vi "Get Current Hour Data ver2.vi"(9 "Shift":string, 10 "Total Hours per Shift":i32=12, 11 "Refnum in":T1) -> (0 "Current Hour Actual":u32, 1 "Hour Index":i32, 2 "Shift Hour Data":u32[][](array[numeric]), 3 "Refnum Out":T1, 4 "Current Hour Target":u32)   [LabVIEW 2018]
uses:
  <vilib>/Utility/config.llb/Config Data RefNum.ctl
  <vilib>/Utility/config.llb/Read Key (String).vi
  <vilib>/Utility/config.llb/NI_LVConfig.lvlib
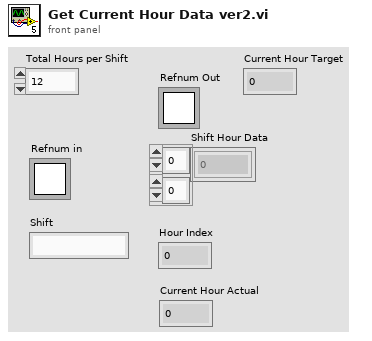
[diagram p1: front panel]
types:
  T1 = typedef "NI_LVConfig.lvlib/Config Data RefNum.ctl" = refnum<k1>
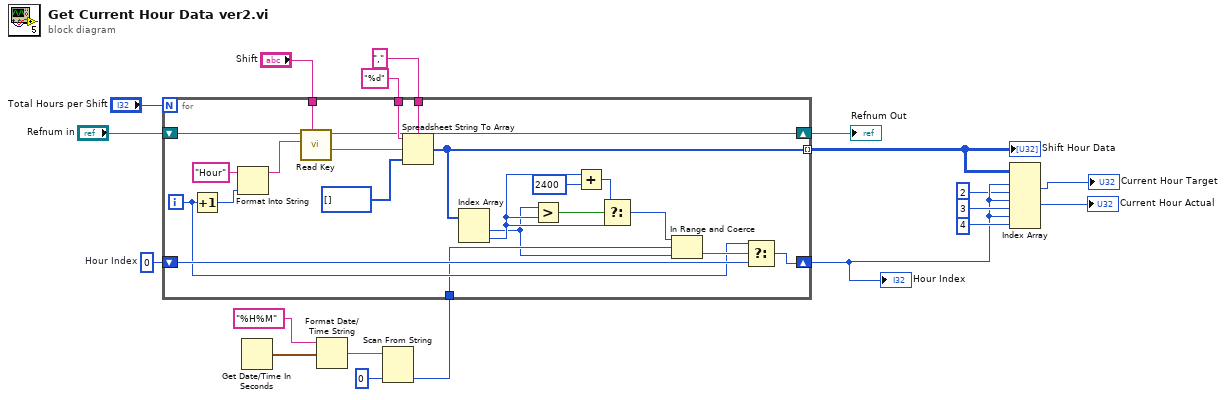
[diagram p0: block diagram]
diagram:
  w16 = 0  # Hour Index
  n1 = Get Date/Time In Seconds() -> (seconds since 1Jan1904=w4:timestamp)
  n2 = Format Date/Time String(time format string (%c)="%H%M", seconds (now)=w4) -> (date/time string=w11:string)  [unwired: 1 in]
  n3 = Scan From String(input string=w11, default 1=u32 0) -> (output 1=w15:u32)  [unwired: 3 in, 3 out]
  n4 = for {
    N: "Total Hours per Shift" -> [_]
    tunnel: "Shift" -> [w41]
    tunnel: [w27] -> w19 mode=indexing
    tunnel: "," ("delimiter (Tab)") -> [w34]
    tunnel: "%d" ("format string") -> [w33]
    tunnel: w15 -> [w28]
    shift-right: [w32] -> w6
    shift-left: w16 -> [w31]
    shift-right: [w26] -> w8
    shift-left: "Refnum in" -> [w40]
    i -> [w29]
    n5 = Increment(x=w29) -> (x+1=w37:i32)
    n6 = Format Into String(initial string="Hour", w37) -> (resulting string=w39:string)  [unwired: 2 in, 1 out]
    n7 = call-poly <vilib>:"Read Key.vi"("section"=w41, "key"=w39, "refnum"=w40) -> ("value"=w36:string, "refnum out"=w26:T1)  [unwired: 5 in, 2 out]
    n8 = Spreadsheet String To Array(delimiter (Tab)=w34, format string=w33, spreadsheet string=w36, array type (2D Dbl)=u32[] []) -> (array=w27:u32[])
    n9 = Index Array(array=w27) -> (element #1=w21:u32, element #2=w22:u32)  [unwired: 2 in]
    n10 = Greater?(x=w21, y=w22) -> (0:w25:bool)
    n11 = Add(x=w22, y=u32 2400) -> (x+y=w23:u32)
    n12 = Select(t=w23, s=w25, f=w22) -> (s? t:f=w20:u32)
    n13 = In Range and Coerce(upper limit=w20, x=w28, lower limit=w21) -> (In Range?=w30:bool)  [unwired: 1 out]
    n14 = Select(t=w29, s=w30, f=w31) -> (s? t:f=w32:i32)
  }
  "Hour Index" <- w6
  "Shift Hour Data" <- w19
  "Refnum Out" <- w8
  n15 = Index Array(array=w19, index (row) #1=w6, index (col) #1=2 ("disabled index (col)"), index (row) #2=w6, index (col) #2=3 ("disabled index (col)"), index (row) #3=w6, index (col) #3=4 ("disabled index (col)")) -> (element #1=→"Current Hour Target":u32, element #2=→"Current Hour Actual":u32)  [unwired: 1 out]
